vi "Catch_nut(show_side).vi"(8 "Error In":errorcluster, 11 "nut_aim":string) -> (0 "Error Out":errorcluster)   [LabVIEW 2019]
uses:
  WSCbot_V3_Toolkit.lvlibp
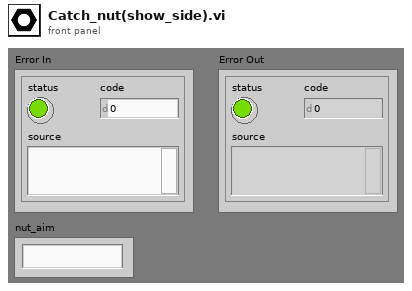
[diagram p1: front panel]
types:
  T1 = enum16{"Right_up", "Right_down", "Left_down", "Left_up", "left", "right", "up", "down"}
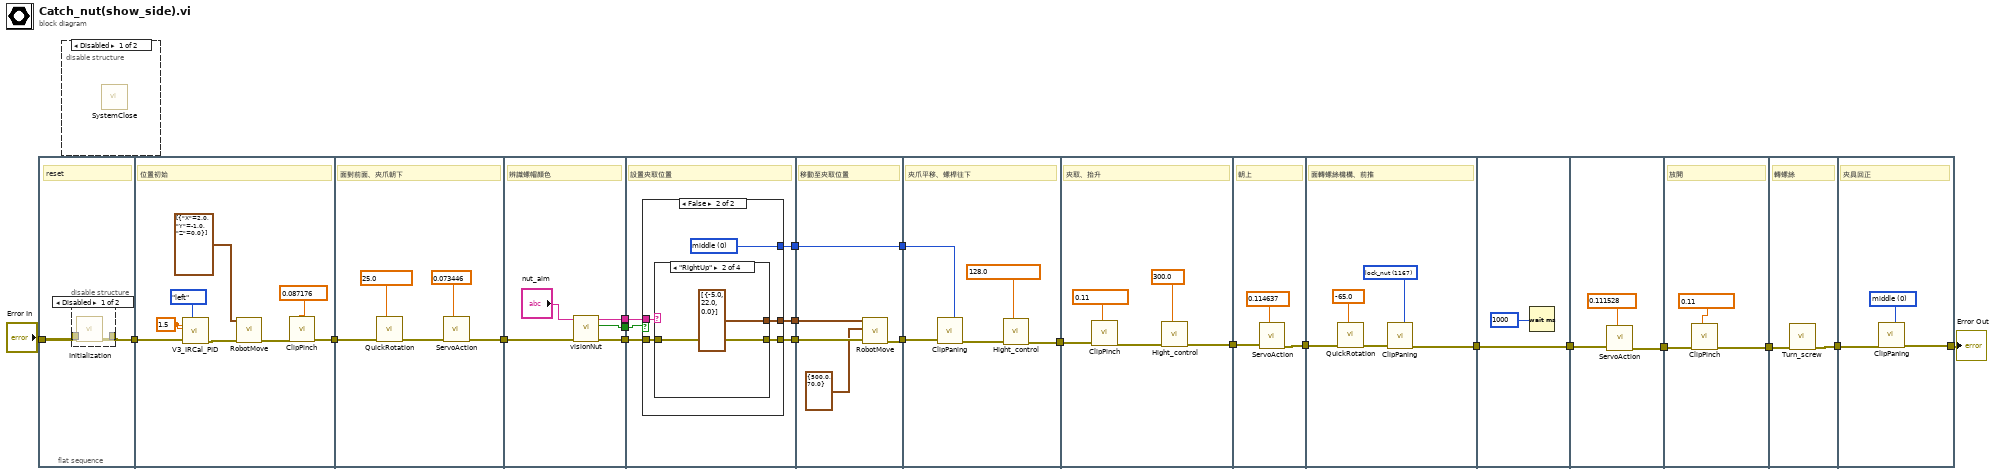
[diagram p0: block diagram]
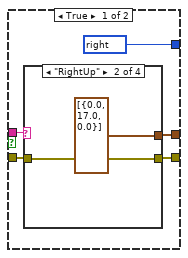
[diagram p4: hidden frame]
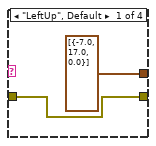
[diagram p5: hidden frame]
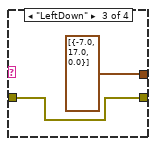
[diagram p6: hidden frame]
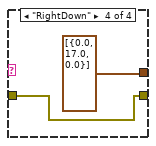
[diagram p7: hidden frame]
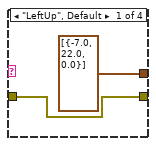
[diagram p8: hidden frame]
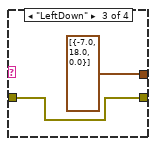
[diagram p9: hidden frame]
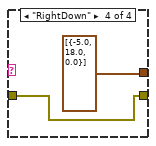
[diagram p10: hidden frame]
diagram:
  n1 = flat-sequence {
    tunnel: "Error In" -> [w23]
    tunnel: [w22] -> w19
    tunnel: [w33] -> w20
    tunnel: w19 -> [w32]
    tunnel: [w36] -> w9
    tunnel: w20 -> [w35]
    tunnel: w9 -> [w43]
    tunnel: [w42] -> w8
    tunnel: [w41] -> w7
    tunnel: [w40] -> w3
    tunnel: w8 -> [w49]
    tunnel: [w48] -> w6
    tunnel: w7 -> [w50]
    tunnel: [w47] -> w4
    tunnel: w3 -> [w46]
    tunnel: [w45] -> w1
    tunnel: w6 -> [w81]
    tunnel: [w80] -> w5
    tunnel: w4 -> [w78]
    tunnel: [w77] -> w2
    tunnel: w1 -> [w77]
    tunnel: w5 -> [w86]
    tunnel: [w84] -> w16
    tunnel: w2 -> [w82]
    tunnel: w16 -> [w90]
    tunnel: [w88] -> w15
    tunnel: [w93] -> w17
    tunnel: w15 -> [w92]
    tunnel: w17 -> [w99]
    tunnel: [w95] -> w12
    tunnel: w12 -> [w101]
    tunnel: [w101] -> w11
    tunnel: [w103] -> w13
    tunnel: w11 -> [w104]
    tunnel: w13 -> [w107]
    tunnel: [w106] -> w14
    tunnel: w14 -> [w108]
    tunnel: [w109] -> w10
    tunnel: [w111] -> w18
    tunnel: w10 -> [w112]
    frame #0 {
      # "reset"
      n2 = disable-structure shown="Disabled" {
        disable-tunnel: w23 -> [w25 w26]
        disable-tunnel: [w24 w26] -> w22
        frame Disabled {
          n3 = call "Initialization.vi"("Error In"=w25) -> ("Error Out"=w24:errorcluster)  [unwired: 10 in]
        }
        frame Enabled {
        }
      }
    }
    frame #1 {
      w27 = 1.5 ("Y_distance(V)")
      w34 = 0.087176 items=["pinch_up"=0.11, "release"=0.087176] ("pinch?")
      # "位置初始"
      n4 = call "V3_IRCal_PID.vi"("Direction"=T1."left", "Error In"=w32, "Y_distance(V)"=w27, "X_distance(V)"=w27) -> ("Error Out"=w30:errorcluster)  [unwired: 6 in, 1 out]
      n5 = call "RobotMove.vi"("error in (no error)"=w30, "XYZ"=cluster{"X":dbl, "Y":dbl, "Z":dbl}[] [{"X"=2.0, "Y"=-1.0, "Z"=0.0}]) -> ("error out"=w29:errorcluster)  [unwired: 9 in]
      n6 = call "ClipPinch.vi"("pinch?"=w34, "Error In"=w29) -> ("Error Out"=w33:errorcluster)  [unwired: 9 in]
    }
    frame #2 {
      w37 = 0.073446 items=["up"=0.1095, "up_up"=0.114637, "down"=0.073446, "back"=0.037435, "back_back"=0.035] ("face_dir")
      w39 = 25.0 items=["Forward"=25.0, "Right"=115.0, "Left"=-65.0] ("螺桿面向")
      # "面對前面、夾爪朝下"
      n7 = call "QuickRotation.vi"("螺桿面向"=w39, "Error In"=w35) -> ("Error Out"=w38:errorcluster)  [unwired: 9 in]
      n8 = call "ServoAction.vi"("face_dir"=w37, "Error In"=w38) -> ("Error Out"=w36:errorcluster)  [unwired: 9 in]
    }
    frame #3 {
      # "辨識螺帽顏色"
      n9 = call "visionNut.vi"("Error In"=w43, "Aim_Color"="nut_aim") -> ("Error Out"=w42:errorcluster, "Left | right"=w40:bool, "Nut_position"=w41:string)  [unwired: 7 in]
    }
    frame #4 {
      # "設置夾取位置"
      n10 = case shown="False" w46 {
        tunnel: w50 -> [w51 w68]
        tunnel: w49 -> [w53 w67]
        tunnel: [w54 w66] -> w48
        tunnel: [w55 w65] -> w47
        tunnel: [w52 w64] -> w45
        frame True {
          w52 = -3500 items=["left"=2100, "right"=-3500, "lock screw"=1345, "middle"=0] ("location")
          n11 = case shown="\"RightUp\"" w51 {
            tunnel: w53 -> [w57 w59 w60 w62]
            tunnel: [w57 w59 w60 w62] -> w54
            tunnel: [cluster{"X":dbl, "Y":dbl, "Z":dbl}[] [{"X"=-7.0, "Y"=17.0, "Z"=0.0}] ("XYZ") cluster{"X":dbl, "Y":dbl, "Z":dbl}[] [{"X"=0.0, "Y"=17.0, "Z"=0.0}] ("XYZ") cluster{"X":dbl, "Y":dbl, "Z":dbl}[] [{"X"=-7.0, "Y"=17.0, "Z"=0.0}] ("XYZ") cluster{"X":dbl, "Y":dbl, "Z":dbl}[] [{"X"=0.0, "Y"=17.0, "Z"=0.0}] ("XYZ")] -> w55
            frame "LeftUp", Default {
            }
            frame "RightUp" {
            }
            frame "LeftDown" {
            }
            frame "RightDown" {
            }
          }
        }
        frame False {
          w64 = 0 items=["left"=2100, "right"=-3500, "lock screw"=1345, "middle"=0] ("location")
          n12 = case shown="\"RightUp\"" w68 {
            tunnel: w67 -> [w70 w72 w73 w75]
            tunnel: [w70 w72 w73 w75] -> w66
            tunnel: [cluster{"X":dbl, "Y":dbl, "Z":dbl}[] [{"X"=-7.0, "Y"=22.0, "Z"=0.0}] ("XYZ") cluster{"X":dbl, "Y":dbl, "Z":dbl}[] [{"X"=-5.0, "Y"=22.0, "Z"=0.0}] ("XYZ") cluster{"X":dbl, "Y":dbl, "Z":dbl}[] [{"X"=-7.0, "Y"=18.0, "Z"=0.0}] ("XYZ") cluster{"X":dbl, "Y":dbl, "Z":dbl}[] [{"X"=-5.0, "Y"=18.0, "Z"=0.0}] ("XYZ")] -> w65
            frame "LeftUp", Default {
            }
            frame "RightUp" {
            }
            frame "LeftDown" {
            }
            frame "RightDown" {
            }
          }
        }
      }
    }
    frame #5 {
      # "移動至夾取位置"
      n13 = call "RobotMove.vi"("error in (no error)"=w81, "Speed/ACC"=cluster{dbl, dbl} {500.0, 70.0}, "XYZ"=w78) -> ("error out"=w80:errorcluster)  [unwired: 8 in]
    }
    frame #6 {
      w83 = 128.0 items=["物料櫃第一格"=0.0, "物料櫃第二格"=78.0, "螺帽夾取高度"=128.0, "螺帽瞄準"=250.0, "最高"=300.0] ("Text Ring")
      # "夾爪平移、螺桿往下"
      n14 = call "ClipPaning.vi"("Error In"=w86, "location"=w82) -> ("Error Out"=w85:errorcluster)  [unwired: 8 in]
      n15 = call "Hight_control.vi"("螺桿高度"=w83, "Error In"=w85) -> ("Error Out"=w84:errorcluster)  [unwired: 9 in]
    }
    frame #7 {
      w87 = 300.0 items=["物料櫃第一格"=0.0, "物料櫃第二格"=78.0, "螺帽夾取高度"=128.0, "螺帽瞄準"=250.0, "最高"=300.0] ("Text Ring")
      w91 = 0.11 items=["pinch_up"=0.11, "release"=0.087176] ("pinch?")
      # "夾取、抬升"
      n16 = call "ClipPinch.vi"("pinch?"=w91, "Error In"=w90) -> ("Error Out"=w89:errorcluster)  [unwired: 9 in]
      n17 = call "Hight_control.vi"("螺桿高度"=w87, "Error In"=w89) -> ("Error Out"=w88:errorcluster)  [unwired: 9 in]
    }
    frame #8 {
      w94 = 0.114637 items=["up"=0.1095, "up_up"=0.114637, "down"=0.073446, "back"=0.037435, "back_back"=0.035] ("face_dir")
      # "朝上"
      n18 = call "ServoAction.vi"("face_dir"=w94, "Error In"=w92) -> ("Error Out"=w93:errorcluster)  [unwired: 9 in]
    }
    frame #9 {
      w96 = 1167 items=["left"=2100, "right"=-3500, "lock screw"=1345, "lock_nut"=1167, "middle"=0] ("location")
      w98 = -65.0 items=["Forward"=25.0, "Right"=115.0, "Left"=-65.0] ("螺桿面向")
      # "面轉螺絲機構、前推"
      n19 = call "QuickRotation.vi"("螺桿面向"=w98, "Error In"=w99) -> ("Error Out"=w97:errorcluster)  [unwired: 9 in]
      n20 = call "ClipPaning.vi"("Error In"=w97, "location"=w96) -> ("Error Out"=w95:errorcluster)  [unwired: 8 in]
    }
    frame #10 {
      n21 = Wait (ms)(milliseconds to wait=u32 1000) -> ()  [unwired: 1 out]
    }
    frame #11 {
      w102 = 0.111528 items=["up"=0.1095, "lock_up"=0.111528, "up_up"=0.114637, "down"=0.073446, "back"=0.037435, "back_back"=0.035] ("face_dir")
      n22 = call "ServoAction.vi"("face_dir"=w102, "Error In"=w104) -> ("Error Out"=w103:errorcluster)  [unwired: 9 in]
    }
    frame #12 {
      w105 = 0.11 items=["pinch_up"=0.11, "release"=0.087176] ("pinch?")
      # "放開"
      n23 = call "ClipPinch.vi"("pinch?"=w105, "Error In"=w107) -> ("Error Out"=w106:errorcluster)  [unwired: 9 in]
    }
    frame #13 {
      # "轉螺絲"
      n24 = call "Turn_screw.vi"("Error In"=w108) -> ("Error Out"=w109:errorcluster)  [unwired: 10 in]
    }
    frame #14 {
      w110 = 0 items=["left"=2100, "right"=-3500, "lock screw"=1345, "lock_nut"=1167, "middle"=0] ("location")
      # "夾具回正"
      n25 = call "ClipPaning.vi"("Error In"=w112, "location"=w110) -> ("Error Out"=w111:errorcluster)  [unwired: 8 in]
    }
  }
  n26 = disable-structure shown="Disabled" {
    frame Disabled {
      n27 = call "SystemClose.vi"() -> ()  [unwired: 3 in, 1 out]
    }
    frame Enabled {
    }
  }
  "Error Out" <- w18
